vi "例9.1 采集一段声音.vi"() -> ()   [LabVIEW 2012]
doc: "本VI说明了从指定设备采集有限声音采样的方式。需要使用连接至声卡的麦克风。可指定需采集的采样数、采样率、通道数和每采样比特率。"
uses:
  <vilib>/sound2/lvsound2.llb/Sampling Mode.ctl
  <vilib>/sound2/lvsound2.llb/Sound Input Read (DBL).vi
panel:
  in  "声音格式":cluster{"采样率(S/s)":dbl, "通道数":dbl, "每采样比特数":dbl}={"采样率(S/s)"=44100.0, "通道数"=2.0, "每采样比特数"=16.0}
  in  "Device ID":u32 caption="设备ID" format="%.0x"
  out "Sound Input":waveform(dbl)[](graph) caption="采集的波形"
  in  "Number of Samples/ch":i32=10000 caption="每通道采样数"
  # "配置"
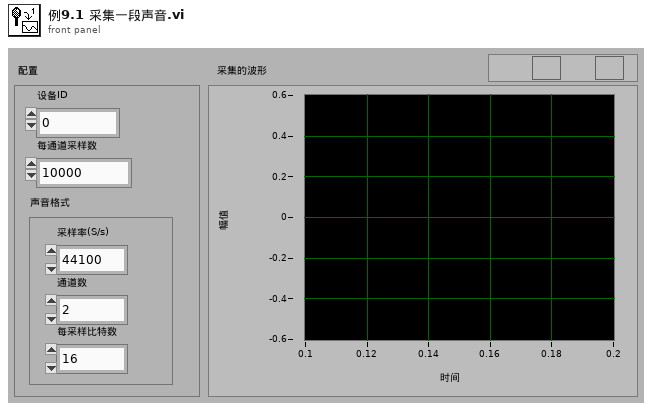
[diagram p1: front panel]
types:
  T1 = typedef "Sampling Mode.ctl" = i32
  T2 = typedef "Sound Input Task ID.ctl" = u32
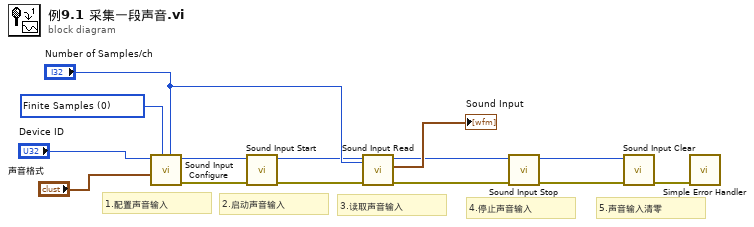
[diagram p0: block diagram]
diagram:
  w12 = T1 0 items=["Finite Samples", "Continuous Samples"] ("sample mode")
  # "5.声音输入清零"
  # "4.停止声音输入"
  # "3.读取声音输入"
  # "2.启动声音输入"
  # "1.配置声音输入"
  n1 = call <vilib>:"Sound Input Configure.vi"("number of samples/ch"="Number of Samples/ch", "sample mode"=w12, "sound format"="声音格式", "device ID"="Device ID") -> ("error out"=w8:errorcluster, "task ID"=w9:T2)  [unwired: 6 in]
  n2 = call <vilib>:"Sound Input Start.vi"("error in (no error)"=w8, "task ID"=w9) -> ("error out"=w6:errorcluster, "task ID out"=w7:T2)  [unwired: 8 in]
  n3 = call-poly <vilib>:"Sound Input Read.vi"("number of samples/ch"="Number of Samples/ch", "error in (no error)"=w6, "task ID"=w7) -> ("error out"=w4:errorcluster, "data"=→"Sound Input":waveform(dbl)[], "task ID out"=w5:T2)  [unwired: 6 in]
  n4 = call <vilib>:"Sound Input Stop.vi"("error in (no error)"=w4, "task ID"=w5) -> ("error out"=w2:errorcluster, "task ID out"=w3:T2)  [unwired: 8 in]
  n5 = call <vilib>:"Sound Input Clear.vi"("error in (no error)"=w2, "task ID"=w3) -> ("error out"=w10:errorcluster)  [unwired: 9 in]
  n6 = call <vilib>:"Simple Error Handler.vi"("error in (no error)"=w10) -> ()  [unwired: 4 in, 5 out]
